vi "close connection.vi"(8 "error in (no error)":errorcluster, 11 "TCP in":refnum<class "TCP.lvclass">) -> (0 "error out":errorcluster, 3 "TCP out":refnum<class "TCP.lvclass">)   [LabVIEW 2021, in "TCP.lvclass"]
doc: "Closes the TCP connection stored in the class."
uses:
  TCP.lvclass
  TCP.lvclass/TCP.ctl
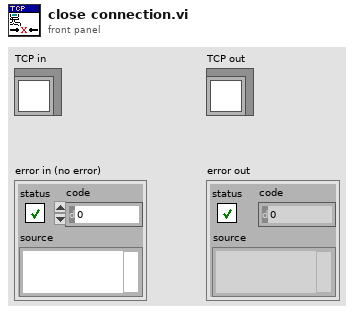
[diagram p1: front panel]
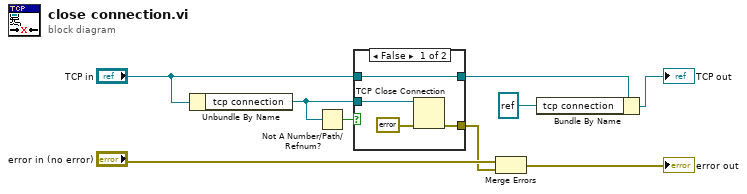
[diagram p0: block diagram]
diagram:
  n1 = Unbundle By Name("TCP in") -> ("tcp connection"=w3:refnum<k5>)
  n2 = Not A Number/Path/Refnum?(number/path/refnum=w3) -> (NaN/Path/Refnum?=w4:bool)
  n3 = case shown="False" w4 {
    tunnel: [w13 _] -> w6
    tunnel: w3 -> [w12 _]
    tunnel: "TCP in" -> [w11 w14]
    tunnel: [w11 w14] -> w1
    frame False {
      n4 = TCP Close Connection(connection ID=w12, error in (no error)=errorcluster {"status"=FALSE, "code"=0, "source"=""}) -> (error out=w13:errorcluster)  [unwired: 1 in, 1 out]
    }
    frame True {
    }
  }
  n5 = Merge Errors("error in (no error)", w6) -> (→"error out":errorcluster)
  n6 = Bundle By Name(cluster=w1, "tcp connection"=refnum<k5> refnum) -> (→"TCP out":refnum<class "TCP.lvclass">)
